vi "KoherasGetSetStatus.vi"() -> ()   [LabVIEW 2013]
panel:
  in  "koheras get set status":cluster{string[], i32[]}
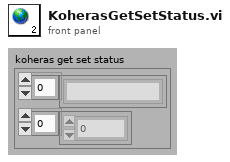
[diagram p1: front panel]
diagram:
